vi "TelegramBOT_Main.vi"() -> ()   [LabVIEW 2014]
uses:
  TelegramBOT_class/SendMsgType.ctl
  TelegramBOT_class/KeyboardMarkup.ctl
  TelegramBOT_class/TelegramBOT.lvclass
panel:
  out "Updates":i32
  out "Msg":i32
  out "Connection":bool
  in  "Stop":bool
  out "error out":errorcluster
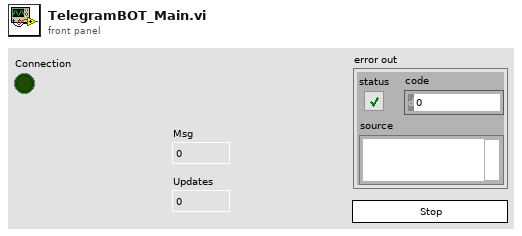
[diagram p1: front panel]
types:
  T1 = typedef "TelegramBOT.lvclass/KeyboardMarkup.ctl" = cluster{"keyboard":cluster{"text":string, "req_loc":bool}[][], "resize_keyboard":bool, "one_time_keyboard":bool, "selective":bool}
  T2 = typedef "TelegramBOT.lvclass/SendMsgType.ctl" = enum16{"Text", "ReplyKeyboardMarkup", "ReplyKeyboardRemove"}
  T3 = typedef "TelegramBOT.lvclass/MessageCluster.ctl" = cluster{"update_id":u32, "from":string, "text":string, "date":timestamp, "chat_id":i32, "type":string, "reply_to_message.text":string, "message_id":u32}
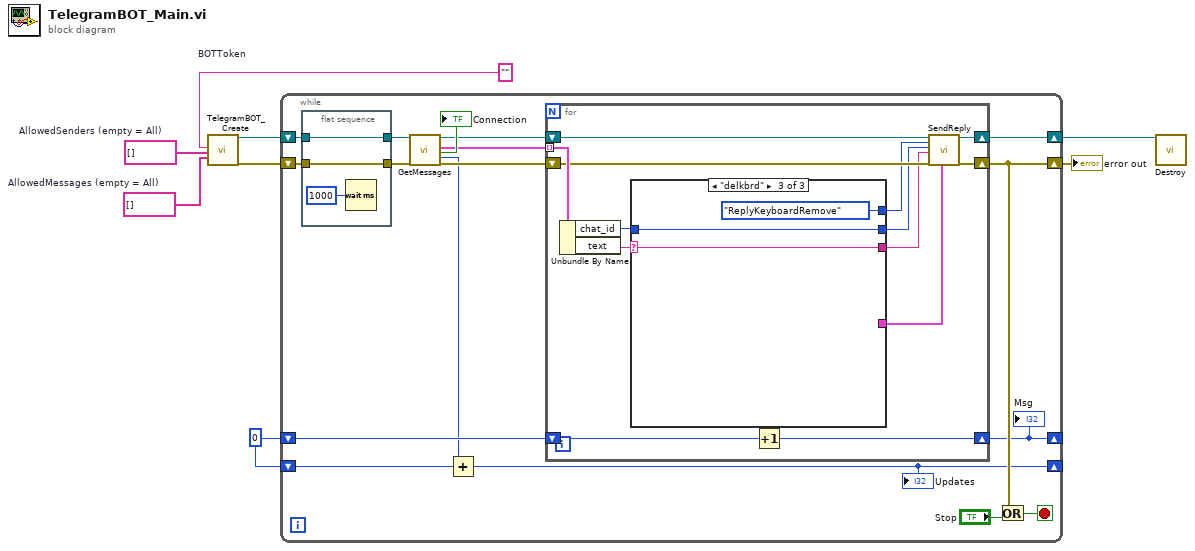
[diagram p0: block diagram]
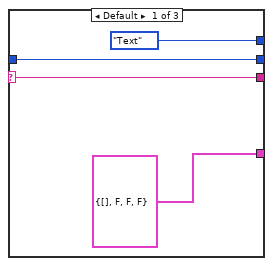
[diagram p2: hidden frame]
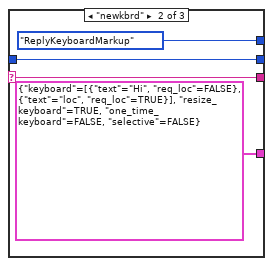
[diagram p3: hidden frame]
diagram:
  w2 = string[] []  # AllowedMessages (empty = All)
  w3 = string[] []  # AllowedSenders (empty = All)
  w1 = 0
  w4 = ""  # BOTToken
  n1 = call "TelegramBOT_Create.vi"("BOTToken"=w4, "AllowedSenders (empty = All)"=w3, "AllowedMessages (empty = All)"=w2) -> ("reference out"=w8:refnum<class "TelegramBOT.lvclass">, "error out"=w6:errorcluster)  [unwired: 15 in]
  n2 = while {
    shift-right: [w15] -> w7
    shift-left: w8 -> [w23]
    shift-right: [w16] -> w5
    shift-left: w6 -> [w22]
    shift-right: [w12] -> _
    shift-left: w1 -> [w13]
    shift-right: [w9] -> _
    shift-left: w1 -> [w10]
    stop <- w25 stop-if-true
    n3 = flat-sequence {
      tunnel: [w52] -> w20
      tunnel: w23 -> [w52]
      tunnel: [w51] -> w21
      tunnel: w22 -> [w51]
      frame #0 {
        n4 = Wait (ms)(milliseconds to wait=u32 1000) -> ()  [unwired: 1 out]
      }
    }
    n5 = call-dynamic "GetMessages.vi"("reference in"=w20, "error in (no error)"=w21) -> ("reference out"=w18:refnum<class "TelegramBOT.lvclass">, "Messages"=w14:T3[], "Connection"=→"Connection":bool, "ReceivedUpdates"=w11:i32, "error out"=w17:errorcluster)  [unwired: 13 in]
    n6 = Add(x=w11, y=w10) -> (x+y=w9:i32)
    "Updates" <- w9
    n7 = for {
      shift-right: [w34] -> w15
      shift-left: w18 -> [w35]
      shift-right: [w32] -> w16
      shift-left: w17 -> [w33]
      tunnel: w14 -> [w38] mode=indexing
      shift-right: [w26] -> w12
      shift-left: w13 -> [w27]
      n8 = Unbundle By Name(w38) -> ("chat_id"=w36:i32, "text"=w37:string)
      n9 = case shown="\"delkbrd\"" w37 {
        selector: w37 -> [w42 w43 w47]
        tunnel: w36 -> [w41 w45 w48]
        tunnel: [w42 w43 w47] -> w31
        tunnel: [w41 w45 w48] -> w30
        tunnel: [SendMsgType."Text" ("MsgType") SendMsgType."ReplyKeyboardMarkup" ("MsgType") SendMsgType."ReplyKeyboardRemove" ("MsgType")] -> w29
        tunnel: [T1 {"keyboard"=[], "resize_keyboard"=FALSE, "one_time_keyboard"=FALSE, "selective"=FALSE} ("ReplyKeyboardMarkup") T1 {"keyboard"=[[{"text"="Hi", "req_loc"=FALSE}], [{"text"="loc", "req_loc"=TRUE}]], "resize_keyboard"=TRUE, "one_time_keyboard"=FALSE, "selective"=FALSE} ("ReplyKeyboardMarkup") _] -> w28
        frame Default {
        }
        frame "newkbrd" {
        }
        frame "delkbrd" {
        }
      }
      n10 = Increment(x=w27) -> (x+1=w26:i32)
      n11 = call-dynamic "SendReply.vi"("reference in"=w35, "MsgType"=w29, "ChatId"=w30, "Text"=w31, "error in (no error)"=w33, "ReplyKeyboardMarkup"=w28) -> ("reference out"=w34:refnum<class "TelegramBOT.lvclass">, "error out"=w32:errorcluster)  [unwired: 12 in]
    }
    "Msg" <- w12
    n12 = Or(x=w16, y="Stop") -> (x .or. y?=w25:bool)
  }
  "error out" <- w5
  n13 = call-dynamic "Destroy.vi"("reference in"=w7) -> ()  [unwired: 17 in, 2 out]
